vi "zadanie_1.vi"() -> ()   [LabVIEW 2020]
panel:
  out "Enum":T1(ring)
  in  "stop":bool
  in  "temp do osiagniecia":dbl min=0.0 step=1.0
  out "pomiar temp":dbl(slide) scale=0.0..100.0
  out "chlodzenie":bool
  out "grzanie":bool
  in  "Boolean 2":bool
  in  "Boolean":bool
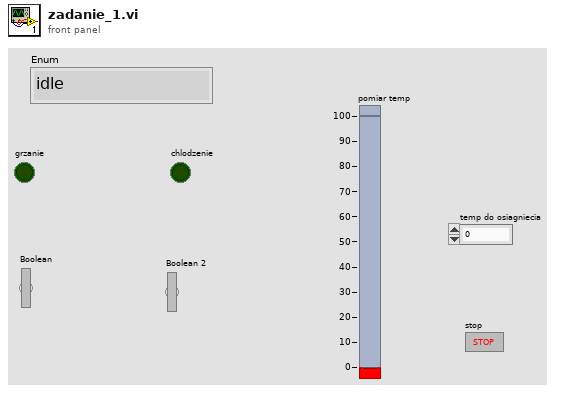
[diagram p1: front panel]
types:
  T1 = enum16{"idle", "odczyt", "grzanie", "chlodzenie"}
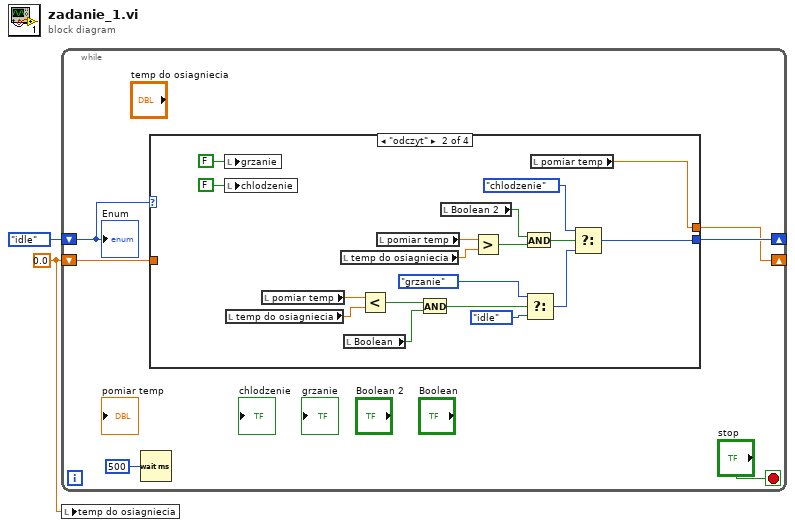
[diagram p0: block diagram]
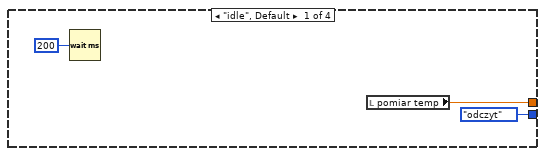
[diagram p2: hidden frame]
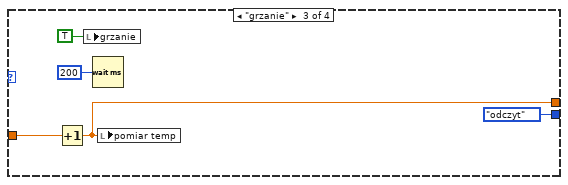
[diagram p3: hidden frame]
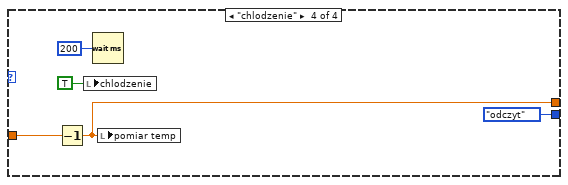
[diagram p4: hidden frame]
diagram:
  w1 = 0.0 ("temp do osiagniecia")
  n1 = while {
    shift-right: [w6] -> _
    shift-left: T1."idle" -> [w5]
    shift-right: [w4] -> _
    shift-left: w1 -> [w3]
    stop <- "stop" stop-if-true
    n2 = Wait (ms)(milliseconds to wait=u32 500) -> ()  [unwired: 1 out]
    n3 = case shown="\"odczyt\"" w5 {
      tunnel: [T1."odczyt" w25 T1."odczyt" T1."odczyt"] -> w6
      tunnel: [w9 w12 w32 w37] -> w4
      tunnel: w3 -> [_ _ w31 w38]
      frame "idle", Default {
        n4 = Wait (ms)(milliseconds to wait=u32 200) -> ()  [unwired: 1 out]
        n5 = local read "pomiar temp"() -> (w9:dbl)
      }
      frame "odczyt" {
        n6 = local write "grzanie"(FALSE ("grzanie")) -> ()
        n7 = local write "chlodzenie"(FALSE ("chlodzenie")) -> ()
        n8 = local read "temp do osiagniecia"() -> (w26:dbl)
        n9 = local read "pomiar temp"() -> (w27:dbl)
        n10 = local read "temp do osiagniecia"() -> (w29:dbl)
        n11 = local read "Boolean"() -> (w20:bool)
        n12 = Less?(x=w27, y=w26) -> (x < y?=w19:bool)
        n13 = local read "pomiar temp"() -> (w28:dbl)
        n14 = And(x=w19, y=w20) -> (x .and. y?=w18:bool)
        n15 = local read "Boolean 2"() -> (w15:bool)
        n16 = Greater?(x=w28, y=w29) -> (0:w17:bool)
        n17 = And(x=w15, y=w17) -> (x .and. y?=w16:bool)
        n18 = Select(t=T1."grzanie", s=w18, f=T1."idle") -> (s? t:f=w24:T1)
        n19 = local read "pomiar temp"() -> (w12:dbl)
        n20 = Select(t=T1."chlodzenie", s=w16, f=w24) -> (s? t:f=w25:T1)
      }
      frame "grzanie" {
        n21 = Increment(x=w31) -> (x+1=w32:dbl)
        n22 = local write "grzanie"(TRUE ("grzanie")) -> ()
        n23 = Wait (ms)(milliseconds to wait=u32 200) -> ()  [unwired: 1 out]
        n24 = local write "pomiar temp"(w32) -> ()
      }
      frame "chlodzenie" {
        n25 = Decrement(x=w38) -> (x-1=w37:dbl)
        n26 = local write "chlodzenie"(TRUE ("chlodzenie")) -> ()
        n27 = Wait (ms)(milliseconds to wait=u32 200) -> ()  [unwired: 1 out]
        n28 = local write "pomiar temp"(w37) -> ()
      }
    }
    "Enum" <- w5
  }
  n29 = local write "temp do osiagniecia"(w1) -> ()
